vi "WheelShooter Aimbot.vi"(1 "input cluster":T10, 2 "Range":dbl) -> (0 "error out":errorcluster)   [LabVIEW 2015]
doc: "Spins up the firing motors and then shoots over one second."
uses:
  <vilib>/Rock Robotics/WPI/MotorControl/WPI_MotorControlDeviceRef.ctl
  <vilib>/Rock Robotics/WPI/MotorControl/WPI_MotorControlType.ctl
  <vilib>/Rock Robotics/SystemInterfaces/DIO/FPGA_DIOPWMChannel.ctl
  <vilib>/Rock Robotics/WPI/PWM/WPI_PWMDeadband.ctl
  <vilib>/Rock Robotics/WPI/CAN/Jaguar/SubVIs/WPI_CANJaguar_ControlMode.ctl
  <vilib>/Rock Robotics/WPI/CAN/TalonSRX/WPI_CANTalonSRX_APIControlMode.ctl
  <vilib>/Rock Robotics/WPI/Solenoid/WPI_SolenoidDevRef.ctl
  <vilib>/Rock Robotics/WPI/Solenoid/WPI_SolenoidChannel.ctl
  <vilib>/Rock Robotics/WPI/Solenoid/WPI_SolenoidValue.ctl
  <vilib>/Rock Robotics/WPI/Solenoid/WPI_SolenoidSetEnum.vi
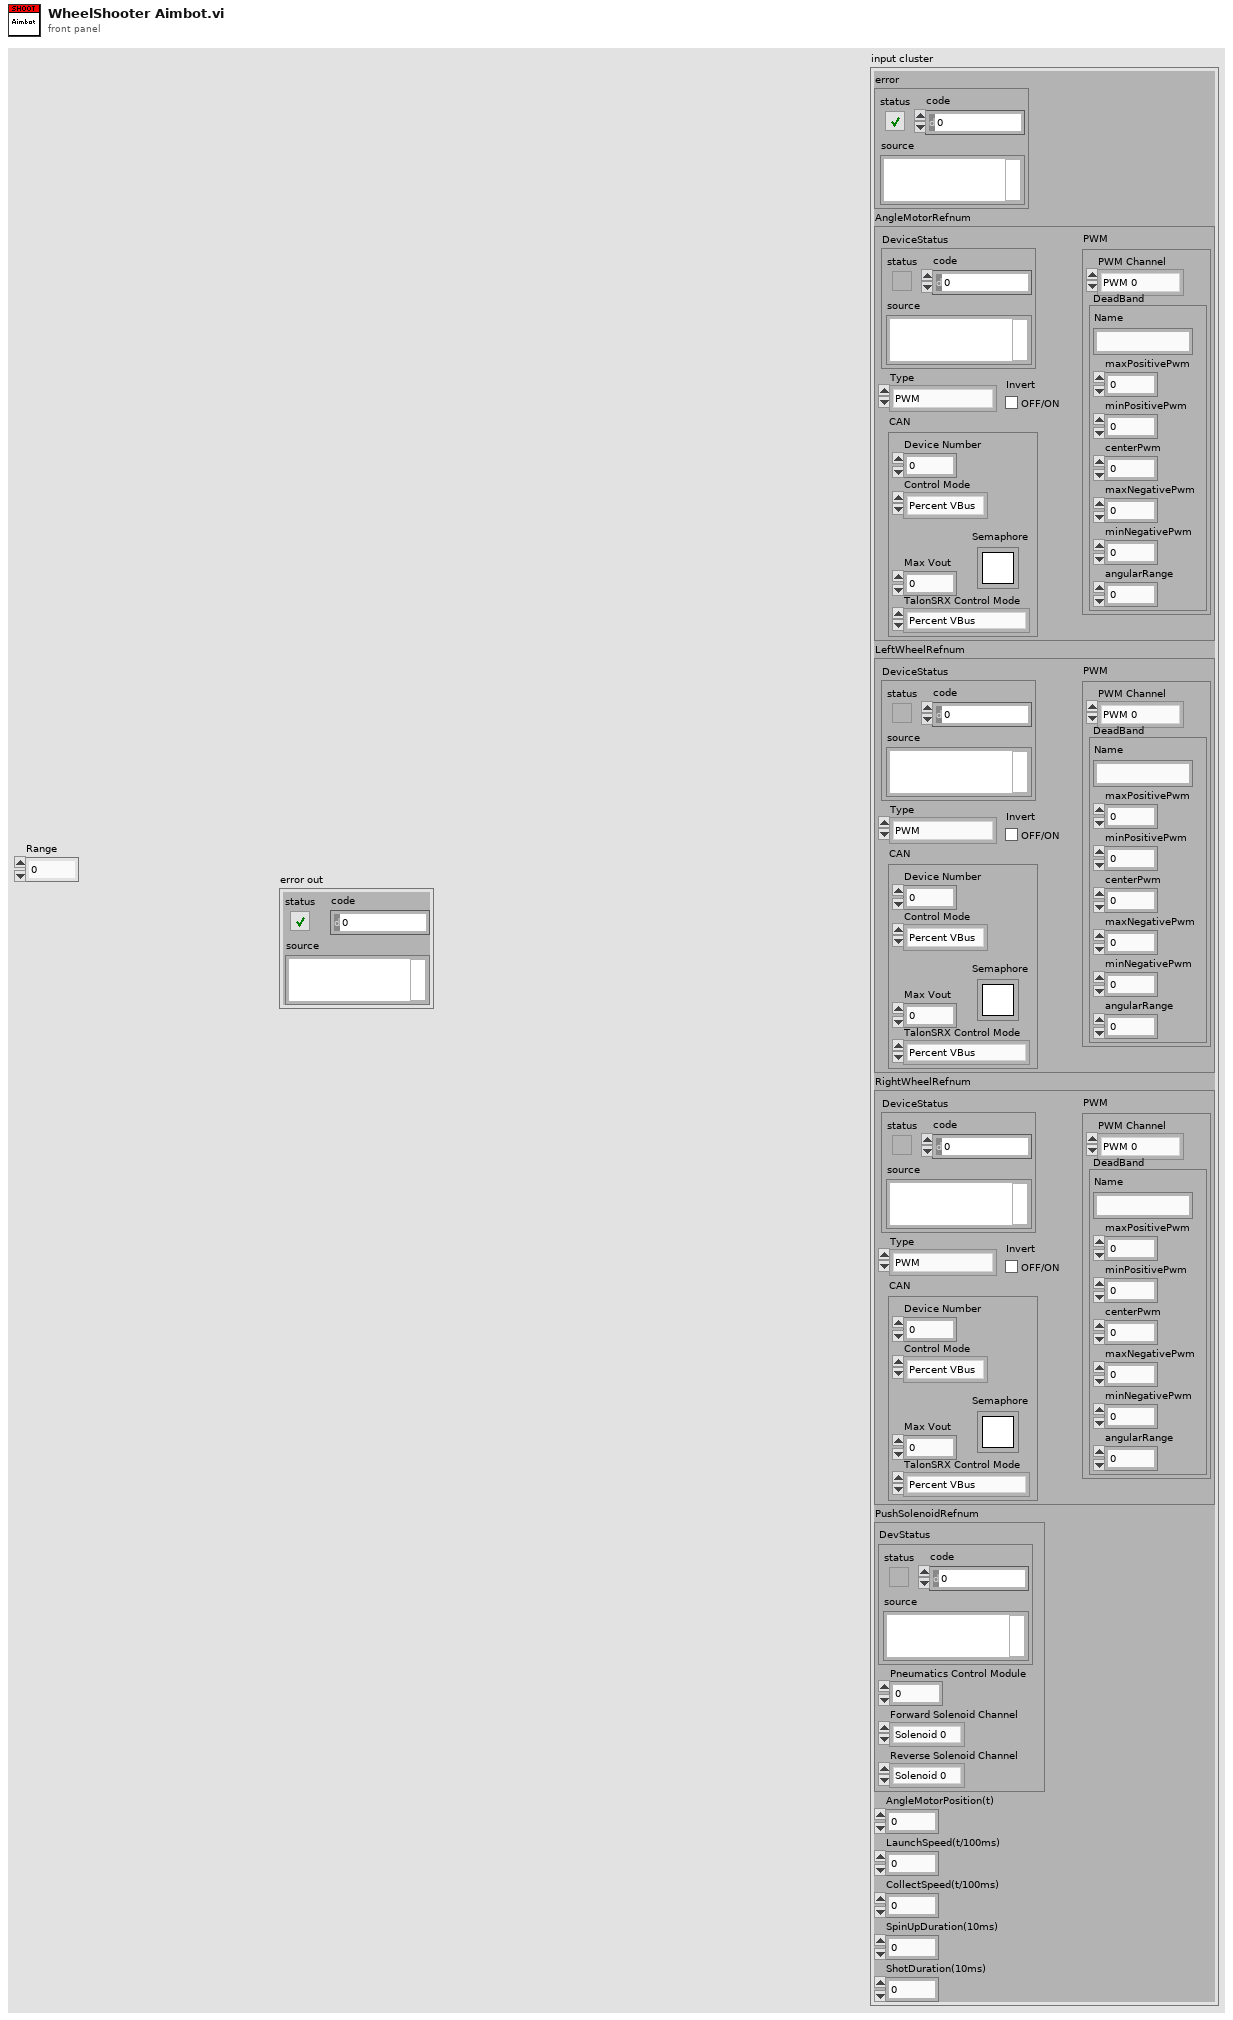
[diagram p1: front panel]
types:
  T1 = typedef "WPI_MotorControlDeviceRef.ctl" = cluster{"DeviceStatus":errorcluster, "Type":T2, "PWM":cluster{"PWM Channel":T3, "DeadBand":T4}, "CAN":cluster{"Device Number":u8, "Control Mode":T5, "Semaphore":T6, "Max Vout":dbl, "TalonSRX Control Mode":T7}, "Invert":bool}
  T2 = typedef "WPI_MotorControlType.ctl" = enum16{"PWM", "CAN", "CANTalonSRX"}
  T3 = typedef "FPGA_DIOPWMChannel.ctl" = enum8{"PWM 0", "PWM 1", "PWM 2", "PWM 3", "PWM 4", "PWM 5", "PWM 6", "PWM 7", "PWM 8", "PWM 9", "PWM MXP 0", "PWM MXP 1", "PWM MXP 2", "PWM MXP 3", "PWM MXP 4", "PWM MXP 5", "PWM MXP 6", "PWM MXP 7", "PWM MXP 8", "PWM MXP 9", "Invalid"}
  T4 = typedef "WPI_PWMDeadband.ctl" = cluster{"Name":string, "maxPositivePwm":i32, "minPositivePwm":i32, "centerPwm":i32, "maxNegativePwm":i32, "minNegativePwm":i32, "angularRange":u16}
  T5 = typedef "WPI_CANJaguar_ControlMode.ctl" = enum8{"Percent VBus", "Current", "Speed", "Position", "Voltage"}
  T6 = typedef "Semaphore RefNum" = refnum<k1>
  T7 = typedef "WPI_CANTalonSRX_APIControlMode.ctl" = enum8{"Percent VBus", "Speed", "Position", "Slave", "Unchanged / Invalid", "Voltage Compensation", "Current", "Motion Profile"}
  T8 = typedef "WPI_SolenoidDevRef.ctl" = cluster{"DevStatus":errorcluster, "Pneumatics Control Module":u8, "Forward Solenoid Channel":T9, "Reverse Solenoid Channel":T9}
  T9 = typedef "WPI_SolenoidChannel.ctl" = enum8{"Solenoid 0", "Solenoid 1", "Solenoid 2", "Solenoid 3", "Solenoid 4", "Solenoid 5", "Solenoid 6", "Solenoid 7", "Invalid"}
  T10 = cluster{"error":errorcluster, "AngleMotorRefnum":T1, "LeftWheelRefnum":T1, "RightWheelRefnum":T1, "PushSolenoidRefnum":T8, "AngleMotorPosition(t)":dbl, "LaunchSpeed(t/100ms)":dbl, "CollectSpeed(t/100ms)":dbl, "SpinUpDuration(10ms)":i32, "ShotDuration(10ms)":i32}
  T11 = typedef "WPI_SolenoidValue.ctl" = enum16{"Off", "On", "Forward", "Reverse"}
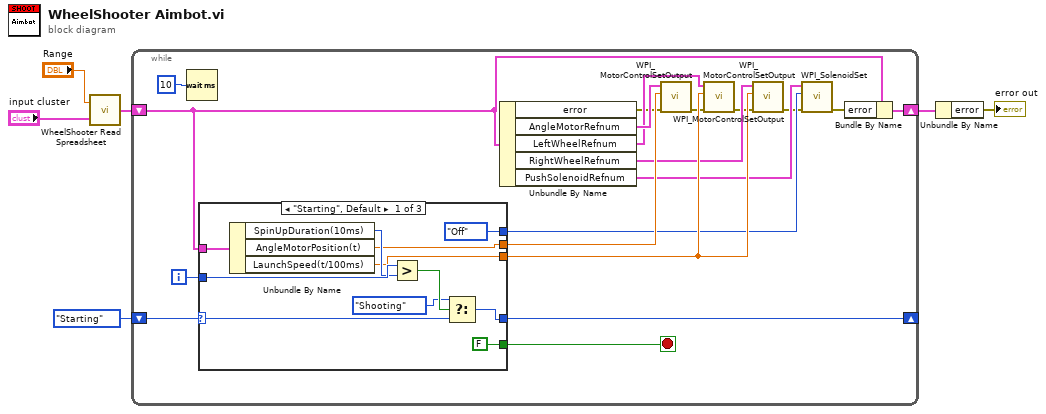
[diagram p0: block diagram]
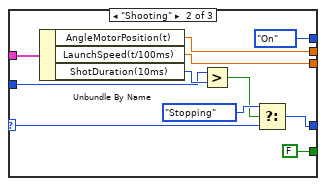
[diagram p2: hidden frame]
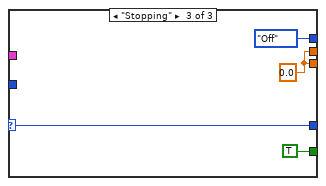
[diagram p3: hidden frame]
diagram:
  n1 = call "WheelShooter Read Spreadsheet.vi"("input cluster"="input cluster", "Range"="Range") -> ("output cluster"=w4:T10)
  n2 = while {
    shift-right: [w22] -> _
    shift-left: enum16{"Starting", "Shooting", "Stopping"}."Starting" -> [w25]
    shift-right: [w16] -> w3
    shift-left: w4 -> [w15]
    i -> [w23]
    stop <- w11 stop-if-true
    n3 = Wait (ms)(milliseconds to wait=u32 10) -> ()  [unwired: 1 out]
    n4 = case shown="\"Starting\", Default" w25 {
      selector: w25 -> [w33 w44 w51]
      tunnel: w23 -> [w36 w45 _]
      tunnel: w15 -> [w35 w47 _]
      tunnel: [w31 w43 w51] -> w22
      tunnel: [w30 w39 w50] -> w21
      tunnel: [w29 w40 w50] -> w20
      tunnel: [FALSE FALSE TRUE] -> w11
      tunnel: [WPI_SolenoidValue."Off" ("Value") WPI_SolenoidValue."On" ("Value") WPI_SolenoidValue."Off" ("Value")] -> w10
      frame "Starting", Default {
        n5 = Unbundle By Name(w35) -> ("SpinUpDuration(10ms)"=w34:i32, "AngleMotorPosition(t)"=w29:dbl, "LaunchSpeed(t/100ms)"=w30:dbl)
        n6 = Greater?(x=w36, y=w34) -> (0:w32:bool)
        n7 = Select(t=enum16{"Starting", "Shooting", "Stopping"}."Shooting", s=w32, f=w33) -> (s? t:f=w31:enum16{"Starting", "Shooting", "Stopping"})
      }
      frame "Shooting" {
        n8 = Unbundle By Name(w47) -> ("AngleMotorPosition(t)"=w40:dbl, "LaunchSpeed(t/100ms)"=w39:dbl, "ShotDuration(10ms)"=w46:i32)
        n9 = Greater?(x=w45, y=w46) -> (0:w41:bool)
        n10 = Select(t=enum16{"Starting", "Shooting", "Stopping"}."Stopping", s=w41, f=w44) -> (s? t:f=w43:enum16{"Starting", "Shooting", "Stopping"})
      }
      frame "Stopping" {
        w50 = 0.0 ("AngleMotorT")
      }
    }
    n11 = Unbundle By Name(w15) -> ("error"=w12:errorcluster, "AngleMotorRefnum"=w19:T1, "LeftWheelRefnum"=w18:T1, "RightWheelRefnum"=w17:T1, "PushSolenoidRefnum"=w9:T8)
    n12 = call <vilib>:"WPI_MotorControlSetOutput.vi"("error in (no error)"=w12, "Output"=w20, "MotorControlDevRef"=w19) -> ("error out"=w13:errorcluster)  [unwired: 6 in, 2 out]
    n13 = call <vilib>:"WPI_MotorControlSetOutput.vi"("error in (no error)"=w13, "Output"=w21, "MotorControlDevRef"=w18) -> ("error out"=w14:errorcluster)  [unwired: 6 in, 2 out]
    n14 = call <vilib>:"WPI_MotorControlSetOutput.vi"("error in (no error)"=w14, "Output"=w21, "MotorControlDevRef"=w17) -> ("error out"=w8:errorcluster)  [unwired: 6 in, 2 out]
    n15 = call-poly <vilib>:"WPI_SolenoidSet.vi"("error in (no error)"=w8, "Value"=w10, "SolenoidDevRef"=w9) -> ("error out"=w7:errorcluster)  [unwired: 7 in, 1 out]
    n16 = Bundle By Name(cluster=w15, "error"=w7) -> (w16:T10)
  }
  n17 = Unbundle By Name(w3) -> ("error"=→"error out":errorcluster)
